vi "Wavelet_Transform.vi"() -> (5 "Plug in titles":string[](array[string]), 7 "Plug in values":string[](array[string]))   [LabVIEW 2010]
uses:
  Globals/Meas_global.vi
  Globals/Plug_in_data_global.vi
panel:
  out "Wavelet plot":dbl[][](graph)
  in  "Full Header Info?":bool
  in  "Time series in First Column?":bool
  in  "Output Directory":path
  in  "Put each block into separate file":bool
  in  "Leave space between blocks?":bool
  in  "Precision":i16=2
  in  "Data to save":i32[](array[ring])=[1] items=["FF (C)"]
  in  "Separation Character":string="\t"
  # "Run this VI to update the channel names"
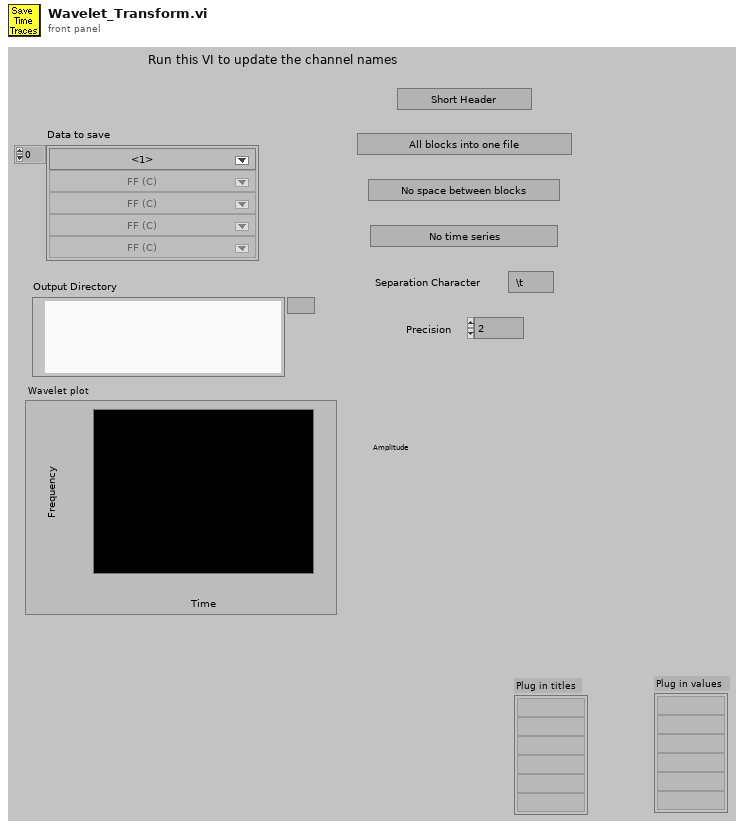
[diagram p1: front panel]
types:
  T1 = typedef "Analysis_info_cluster.ctl" = cluster{"Colour":u32, "Inst type":T2, "Inst name":string, "Symbol":string, "Code name":string, "Extra Info":string, "Inst Array":T3, "Index":i32, "Voltage Index":i32, "Extra Titles":string[], "Extra Values":string[]}
  T2 = typedef "Inst_type.ctl" = enum16{"Propeller anemometer", "Raw voltage", "Pressure Transducer", "Pitot-static tube", "Preston tube", "Hot wire", "Cross wire 1", "Cross wire 2", "Generic Linear", "Generic Polynomial", "Generic BackPoly", "Fast FID", "Thermocouple", "Cold wire", "Pulsed Wire", "LDA Vel", "LDA Tran time", "LDA Arr time"}
  T3 = typedef "Instrument_Array.ctl" = enum16{"PWA", "LDA", "Analogue"}
  T4 = enum32{"existing file", "new file", "new or existing file", "existing dir", "new dir", "new or existing dir", "existing file (use LLBs)", "new file (use LLBs)", "new or existing file (use LLBs)", "new or existing file or directory (use LLBs)"}
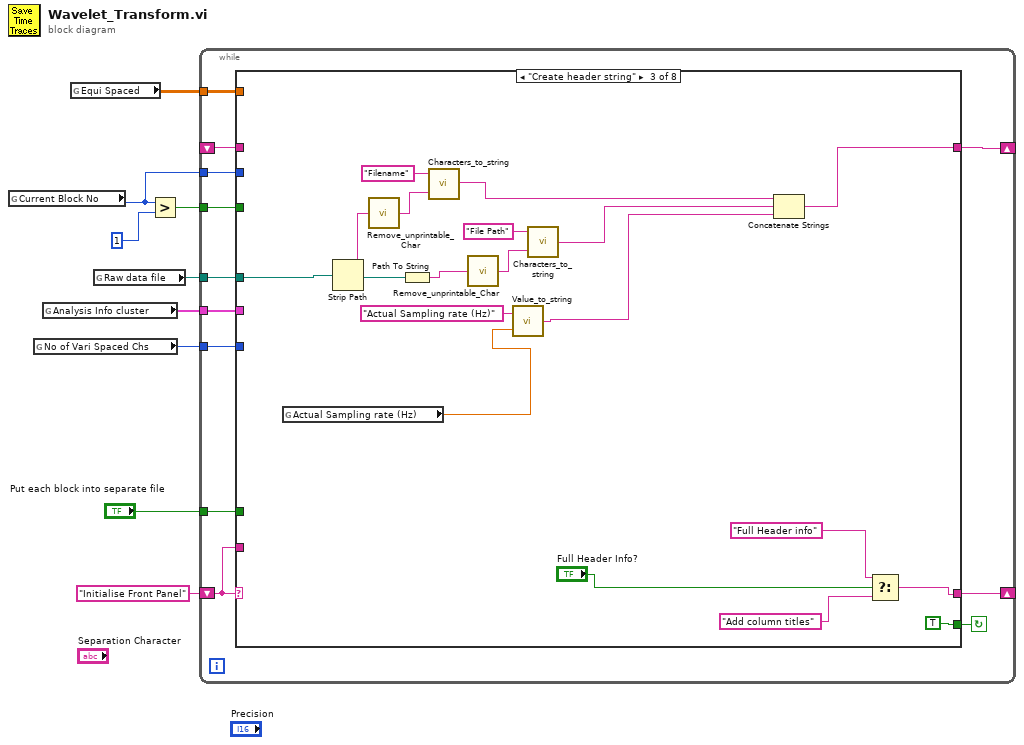
[diagram p0: block diagram]
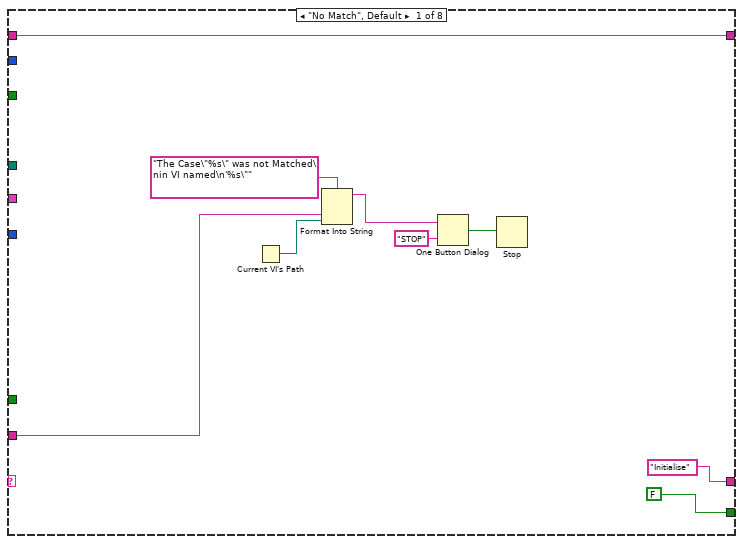
[diagram p2: hidden frame]
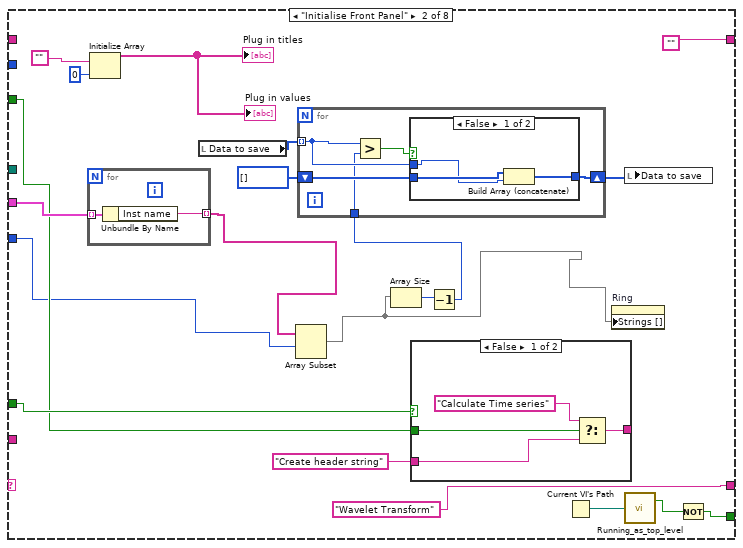
[diagram p3: hidden frame]
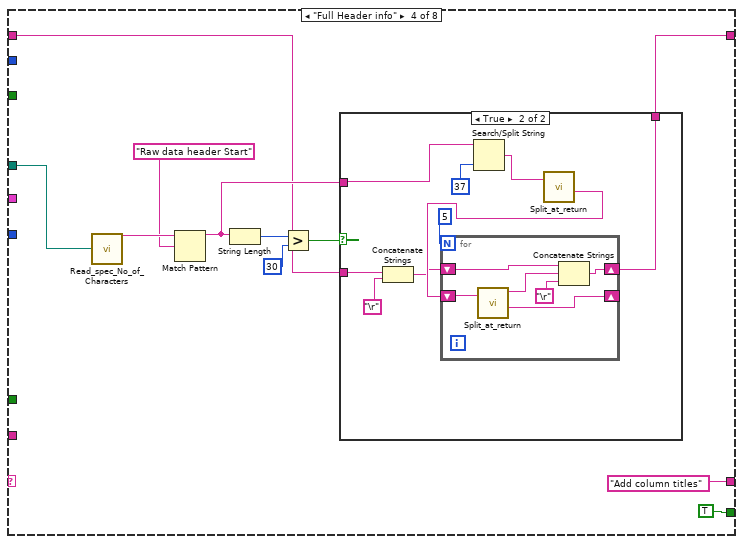
[diagram p6: hidden frame]
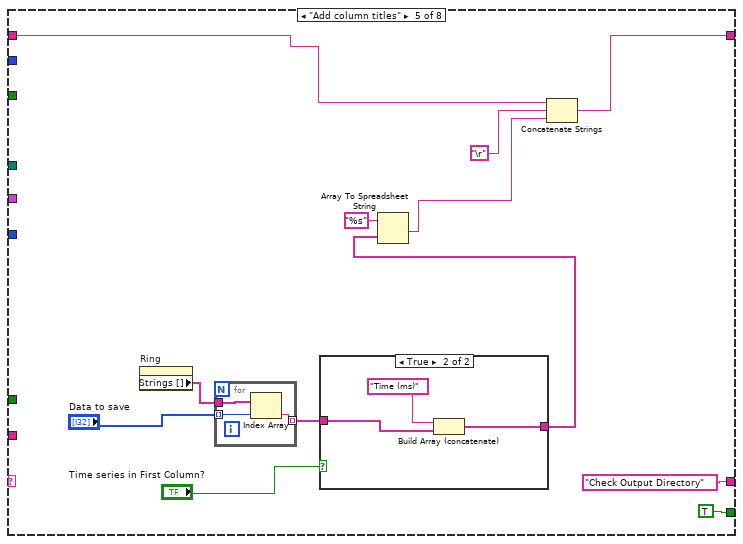
[diagram p8: hidden frame]
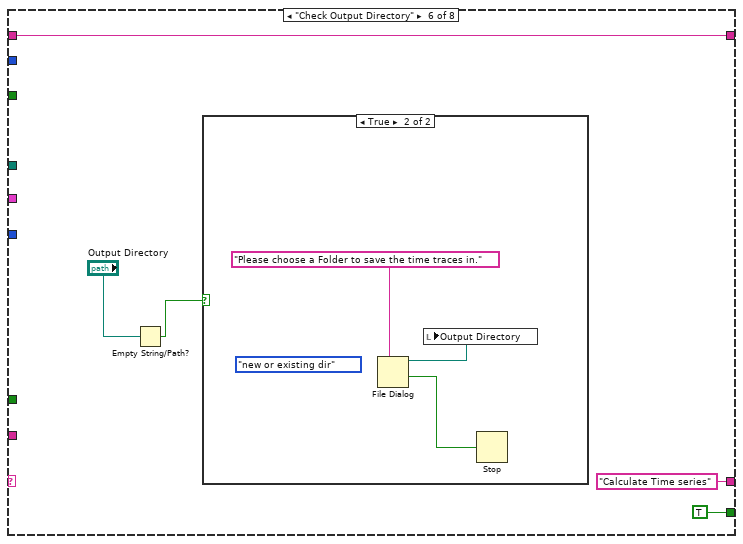
[diagram p10: hidden frame]
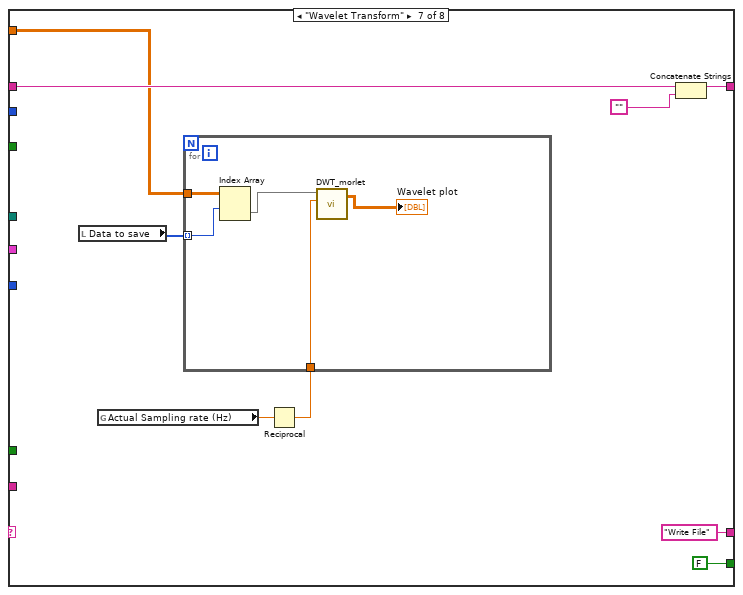
[diagram p12: hidden frame]
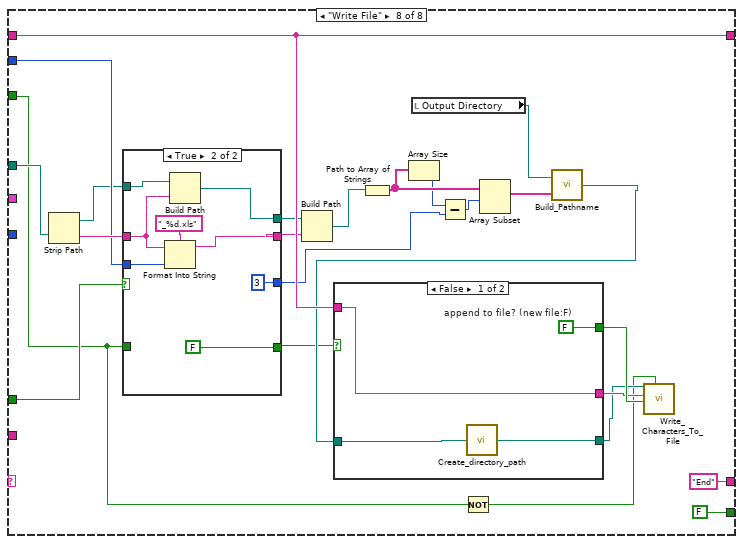
[diagram p13: hidden frame]
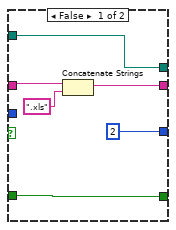
[diagram p14: hidden frame]
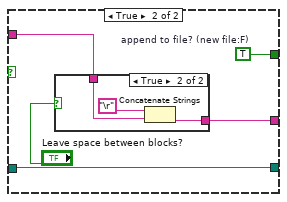
[diagram p15: hidden frame]
diagram:
  n1 = global read "Meas_global.vi" "Current Block No"() -> (w4:i32)
  n2 = global read "Meas_global.vi" "No of Vari Spaced Chs"() -> (w2:i32)
  n3 = global read "Meas_global.vi" "Analysis Info cluster"() -> (w3:T1[])
  n4 = global read "Plug_in_data_global.vi" "Equi Spaced"() -> (w1:dbl[][])
  n5 = global read "Meas_global.vi" "Raw data file"() -> (w7:path)
  n6 = Greater?(x=w4, y=1) -> (0:w5:bool)
  n7 = while {
    shift-left: "Initialise Front Panel" -> [w19]
    shift-right: [w20] -> _
    shift-right: [w16] -> _
    shift-left: _ -> [w15]
    tunnel: "Put each block into separate file" -> [w18]
    tunnel: w7 -> [w17]
    tunnel: w5 -> [w14]
    tunnel: w4 -> [w13]
    tunnel: w3 -> [w12]
    tunnel: w2 -> [w11]
    tunnel: w1 -> [w10]
    stop <- w21 continue-if-true
    n8 = case shown="\"Create header string\"" w19 {
      tunnel: [FALSE w42 TRUE TRUE TRUE TRUE FALSE FALSE] -> w21
      tunnel: ["Initialise" "Wavelet Transform" w67 "Add column titles" ("t") "Check Output Directory" ("t") "Calculate Time series" ("t") "Write File" "End" ("t")] -> w20
      tunnel: w19 -> [w25 _ _ _ _ _ _ _]
      tunnel: w18 -> [_ w40 _ _ _ _ _ w160]
      tunnel: w17 -> [_ _ w75 w89 _ _ _ w176]
      tunnel: [w22 "" w74 w88 w121 w134 w147 w172] -> w16
      tunnel: w15 -> [w22 _ _ w87 w115 w134 w148 w172]
      tunnel: w14 -> [_ w39 _ _ _ _ _ w154]
      tunnel: w13 -> [_ _ _ _ _ _ _ w162]
      tunnel: w12 -> [_ w46 _ _ _ _ _ _]
      tunnel: w11 -> [_ w33 _ _ _ _ _ _]
      tunnel: w10 -> [_ _ _ _ _ _ w143 _]
      frame "No Match", Default {
        n9 = Current VI's Path() -> (path=w24:path)
        n10 = Format Into String(format string="The Case\"%s\" was not Matched\nin VI named\n'%s\"" ("Format String"), w25, w24) -> (resulting string=w28:string)  [unwired: 2 in, 1 out]
        n11 = One Button Dialog(message=w28, button name ("OK")="STOP") -> (true=w26:bool)
        n12 = Stop(stop? (T)=w26) -> ()
      }
      frame "Initialise Front Panel" {
        n13 = for {
          tunnel: w46 -> [w66] mode=indexing
          tunnel: [w65] -> w36 mode=indexing
          n14 = Unbundle By Name(w66) -> ("Inst name"=w65:string)
        }
        n15 = Initialize Array("", 0) -> (→"Plug in values" →"Plug in titles":string[])
        n16 = local read "Data to save"() -> (w45:i32[])
        n17 = Array Subset(array=w36, index=w33) -> (w32:string[])  [unwired: 1 in]
        n18 = Array Size(array=w32) -> (size(s)=w35:i32)
        n19 = case shown="False" w40 {
          tunnel: [w54 w55] -> _
          tunnel: w39 -> [w53 _]
          tunnel: "Create header string" -> [w51 w55]
          frame False {
            n20 = Select(t="Calculate Time series", s=w53, f=w51) -> (s? t:f=w54:string)
          }
          frame True {
          }
        }
        n21 = Decrement(x=w35) -> (x-1=w34:i32)
        n22 = for {
          tunnel: w45 -> [w57] mode=indexing
          shift-right: [w58] -> w43
          shift-left: i32[] [] -> [w59]
          tunnel: w34 -> [w56]
          n23 = Greater?(x=w57, y=w56) -> (0:w60:bool)
          n24 = case shown="False" w60 {
            tunnel: w59 -> [w63 w64]
            tunnel: [w62 w64] -> w58
            tunnel: w57 -> [w61 _]
            frame False {
              n25 = Build Array (concatenate)(w63, w61) -> (w62:i32[])
            }
            frame True {
            }
          }
        }
        n26 = Current VI's Path() -> (path=w38:path)
        n27 = property on="Ring" class="Ring (strict)"("Strings []"=w32) -> ()  [unwired: 2 in, 2 out]
        n28 = local write "Data to save"(w43) -> ()
        n29 = call "Running_as_top_level.vi"("Vi path name"=w38) -> ("Top Level"=w37:bool)  [unwired: 1 out]
        n30 = Not(x=w37) -> (.not. x?=w42:bool)
      }
      frame "Create header string" {
        n31 = global read "Meas_global.vi" "Actual Sampling rate (Hz)"() -> (w71:dbl)
        n32 = Strip Path(path=w75) -> (stripped path=w81:path, name=w77:string)
        n33 = call "Remove_unprintable_Char.vi"("Input String"=w77) -> ("Output String"=w78:string)
        n34 = Path To String(path=w81) -> (string=w82:string)
        n35 = call "Characters_to_string.vi"("Characters to write"=w78, "Label for characters"="Filename") -> ("Output string"=w83:string)
        n36 = call "Remove_unprintable_Char.vi"("Input String"=w82) -> ("Output String"=w79:string)
        n37 = call "Value_to_string.vi"("Value"=w71, "Label for value"="Actual Sampling rate (Hz)") -> ("Output string"=w72:string)  [unwired: 1 in]
        n38 = call "Characters_to_string.vi"("Characters to write"=w79, "Label for characters"="File Path") -> ("Output string"=w84:string)
        n39 = Concatenate Strings(w83, w84, w72) -> (w74:string)
        n40 = Select(t="Full Header info", s="Full Header Info?", f="Add column titles" ("t")) -> (s? t:f=w67:string)
      }
      frame "Full Header info" {
        n41 = call "Read_spec_No_of_Characters.vi"("Filename"=w89) -> ("character string"=w95:string)  [unwired: 1 out]
        n42 = Match Pattern(string=w95, regular expression="Raw data header Start") -> (before substring=w91:string)  [unwired: 4 out]
        n43 = String Length(string=w91) -> (length=w90:i32)
        n44 = Greater?(x=w90, y=30) -> (0:w92:bool)
        n45 = case shown="True" w92 {
          tunnel: w91 -> [_ w105]
          tunnel: w87 -> [w97 w100]
          tunnel: [w97 w103] -> w88
          frame False {
          }
          frame True {
            n46 = Concatenate Strings(w100, "\r") -> (w99:string)
            n47 = Search/Split String(string=w105, offset (0)=37 ("y")) -> (match + rest of string=w102:string)  [unwired: 3 out]
            n48 = call "Split_at_return.vi"("String"=w102) -> ("after substring"=w101:string)  [unwired: 1 in, 3 out]
            n49 = for {
              N: 5 -> [_]
              shift-right: [w110] -> w103
              shift-left: w99 -> [w112]
              shift-right: [w108] -> _
              shift-left: w101 -> [w109]
              n50 = call "Split_at_return.vi"("String"=w109) -> ("before substring"=w111:string, "after substring"=w108:string)  [unwired: 1 in, 2 out]
              n51 = Concatenate Strings(w112, w111, "\r") -> (w110:string)
            }
          }
        }
      }
      frame "Add column titles" {
        n52 = property on="Ring" class="Ring (strict)"() -> ("Strings []"=w117:string[])  [unwired: 2 in, 2 out]
        n53 = for {
          tunnel: w117 -> [w127]
          tunnel: "Data to save" -> [w126] mode=indexing
          tunnel: [w125] -> w116 mode=indexing
          n54 = Index Array(array=w127, index=w126) -> (element=w125:string)
        }
        n55 = case shown="True" "Time series in First Column?" {
          tunnel: w116 -> [w128 w131]
          tunnel: [w128 w130] -> w123
          frame False {
          }
          frame True {
            n56 = Build Array (concatenate)("Time (ms)", w131) -> (w130:string[])
          }
        }
        n57 = Array To Spreadsheet String(array=w123, 3:"%s" ("format string")) -> (spreadsheet string=w118:string)  [unwired: 1 out]
        n58 = Concatenate Strings(w115, "\r", w118) -> (w121:string)
      }
      frame "Check Output Directory" {
        n59 = Empty String/Path?(string/path="Output Directory") -> (empty?=w135:bool)
        n60 = case shown="True" w135 {
          frame False {
          }
          frame True {
            (unwired) T4."new or existing dir" ("select mode (2)")
            n61 = File Dialog(7:"Please choose a Folder to save the time traces in." ("prompt")) -> (1:w138:bool, 3:w139:path)  [unwired: 1 in, 7 out]
            n62 = local write "Output Directory"(w139) -> ()
            n63 = Stop(stop? (T)=w138) -> ()
          }
        }
      }
      frame "Wavelet Transform" {
        n64 = local read "Data to save"() -> (w144:i32[])
        n65 = global read "Meas_global.vi" "Actual Sampling rate (Hz)"() -> (w141:dbl)
        n66 = Reciprocal(x=w141) -> (1/x=w140:dbl)
        n67 = for {
          tunnel: w144 -> [w152] mode=indexing
          tunnel: w143 -> [w153]
          tunnel: w140 -> [w150]
          n68 = Index Array(array=w153, index (row)=w152) -> (element=w151:dbl[])  [unwired: 1 in]
          n69 = call "DWT_morlet.vi"("dt"=w150, "1D Real input"=w151) -> ("Wavelet plot"=→"Wavelet plot":dbl[][])  [unwired: 5 out]
        }
        n70 = Concatenate Strings(w148, "") -> (w147:string)
      }
      frame "Write File" {
        n71 = Strip Path(path=w176) -> (stripped path=w157:path, name=w163:string)
        n72 = case shown="True" w160 {
          tunnel: w163 -> [w183 w186]
          tunnel: w162 -> [_ w191]
          tunnel: [w182 w189] -> w161
          tunnel: w154 -> [w180 _]
          tunnel: [w180 FALSE] -> w159
          tunnel: [w179 w185] -> w158
          tunnel: w157 -> [w179 w187]
          tunnel: [2 ("y") 3 ("y")] -> w156
          frame False {
            n73 = Concatenate Strings(w183, ".xls" ("string")) -> (w182:string)
          }
          frame True {
            n74 = Format Into String(format string="_%d.xls", initial string=w186, w191) -> (resulting string=w189:string)  [unwired: 1 in, 1 out]
            n75 = Build Path(base path=w187, name or relative path=w186) -> (appended path=w185:path)
          }
        }
        n76 = Build Path(base path=w158, name or relative path=w161) -> (appended path=w177:path)
        n77 = Path to Array of Strings(0:w177) -> (2:w169:string[])  [unwired: 1 out]
        n78 = Array Size(array=w169) -> (size(s)=w168:i32)
        n79 = local read "Output Directory"() -> (w165:path)
        n80 = Subtract(x=w168, y=w156) -> (x-y=w167:i32)
        n81 = Not(x=w154) -> (.not. x?=w155:bool)
        n82 = Array Subset(array=w169, index=w167) -> (w166:string[])  [unwired: 1 in]
        n83 = call "Build_Pathname.vi"("Output Array"=w166, "Pathname"=w165) -> ("Appended path"=w164:path)
        n84 = case shown="False" w159 {
          tunnel: [w192 w200] -> w174
          tunnel: w172 -> [w192 w199]
          tunnel: [w195 w198] -> w175
          tunnel: w164 -> [w194 w196]
          tunnel: [w193 w196] -> w173
          frame False {
            w195 = FALSE  # append to file? (new file:F)
            n85 = call "Create_directory_path.vi"("Path name"=w194) -> ("Path name Out"=w193:path)
          }
          frame True {
            w198 = TRUE  # append to file? (new file:F)
            n86 = case shown="True" "Leave space between blocks?" {
              tunnel: [w201 w204] -> w200
              tunnel: w199 -> [w201 w203]
              frame False {
              }
              frame True {
                n87 = Concatenate Strings("\r", w203) -> (w204:string)
              }
            }
          }
        }
        n88 = call "Write_Characters_To_File.vi"("file path (dialog if empty)"=w173, "advisory dialog? (display:T)"=w155, "character string"=w174, "append to file? (new file:F)"=w175) -> ()  [unwired: 1 in, 4 out]
      }
    }
  }
